vi "refmgr_unRegister.vi"(8 "error in (no error)":errorcluster, 10 "Key":string, 11 "TagDB in":T1) -> (0 "error out":errorcluster, 3 "TagDB out":T1)   [LabVIEW 2014, in "RefManager(dev).lvlib"]
uses:
  RefManager(dev).lvlib
  <userlib>/_NEVSTOP/TagDB/Core/tagDB_Def.ctl
  <userlib>/_NEVSTOP/TagDB/Core/_Support/Error/_Clear Errors.vi
  <userlib>/_NEVSTOP/TagDB/Core/_Support/Properties/tagDB dbChanged.vi
  <userlib>/_NEVSTOP/TagDB/Core/_Support/Properties/tagDB getTags.vi
  <userlib>/_NEVSTOP/TagDB/Core/_Support/Access/_variant.vi
  <userlib>/_NEVSTOP/TagDB/Core/_XNode/tagDB_value.xnode/tagDB_value.xnode
  <userlib>/_NEVSTOP/TagDB/Core/TagDB.lvlib
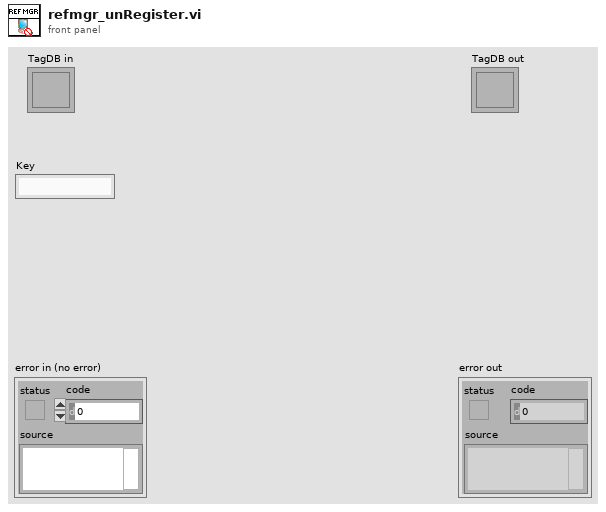
[diagram p1: front panel]
types:
  T1 = typedef "TagDB.lvlib/tagDB_Def.ctl" = refnum<k1>
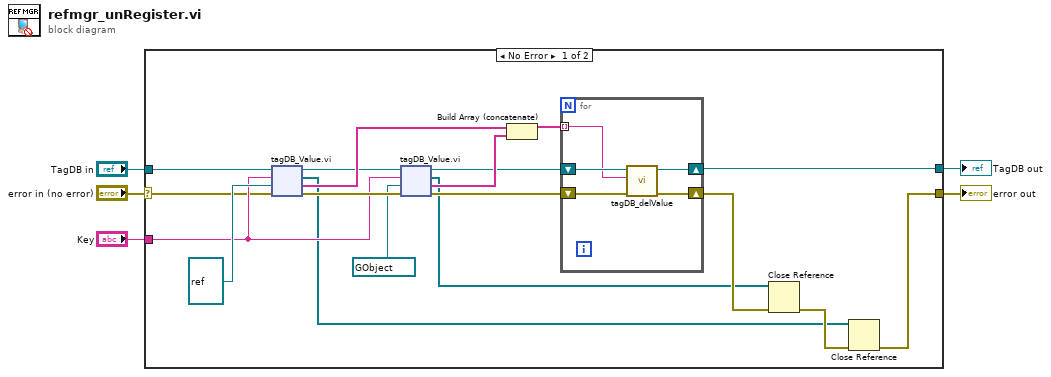
[diagram p0: block diagram]
diagram:
  n1 = case shown="No Error" "error in (no error)" {
    selector: "error in (no error)" -> [w12 w228]
    tunnel: [w23 w228] -> w4
    tunnel: [w10 w227] -> w2
    tunnel: "TagDB in" -> [w13 w227]
    tunnel: "Key" -> [w17 _]
    frame No Error {
      n2 = xnode "tagDB_Value.vi"("error in (no error)"=w12, "DB Ref"=w13, "Type"=refnum<vi> refnum ("VI out"), "RegExp"=w17) -> ("error out"=w19:errorcluster, "DB Ref(dup)"=w20:T1, "value"=w6:refnum<vi>[], "names"=w22:string[])
      n3 = xnode "tagDB_Value.vi"("error in (no error)"=w19, "DB Ref"=w20, "Type"=refnum<vi> refnum, "RegExp"=w17) -> ("error out"=w18:errorcluster, "DB Ref(dup)"=w11:T1, "value"=w7:refnum<vi>[], "names"=w14:string[])
      n4 = Build Array (concatenate)(w22, w14) -> (w15:string[])
      n5 = for {
        tunnel: w15 -> [w222] mode=indexing
        shift-right: [w225] -> w10
        shift-left: w11 -> [w226]
        shift-right: [w224] -> w8
        shift-left: w18 -> [w223]
        n6 = call <userlib>:"tagDB_delValue.vi"("error in (no error)"=w223, "name"=w222, "DB Ref"=w226) -> ("error in (no error) (dup)"=w224:errorcluster, "DB Ref (dup)"=w225:T1)  [unwired: 7 in]
      }
      n7 = Close Reference(reference=w7, error in (no error)=w8) -> (error out=w9:errorcluster)
      n8 = Close Reference(reference=w6, error in (no error)=w9) -> (error out=w23:errorcluster)
    }
    frame Error {
    }
  }
  "error out" <- w4
  "TagDB out" <- w2
